vi "Check Length.vi"(7 "source vi name":string, 8 "error in (no error)":errorcluster, 9 "offset (0)":u64 format="%d bytes", 10 "length (-1: rest)":i64=-1 format="%d bytes", 11 "Pointer in":refnum<class "Pointer.lvclass">) -> (0 "error out":errorcluster, 1 "offset":u64 format="%d bytes", 2 "size":u64 format="%d bytes", 3 "Pointer out":refnum<class "Pointer.lvclass">)   [LabVIEW 2027, in "Memory Manager.lvlib" / "Pointer.lvclass"]
uses:
  Pointer.lvclass
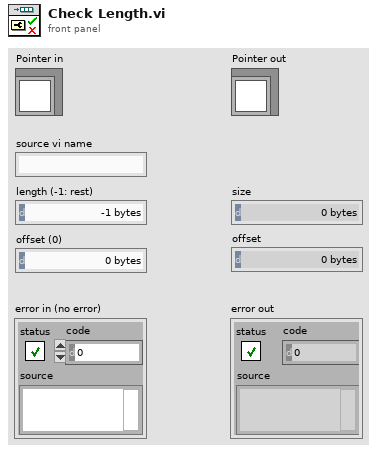
[diagram p1: front panel]
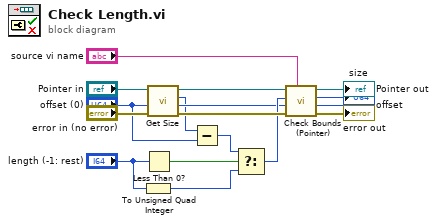
[diagram p0: block diagram]
diagram:
  n1 = To Unsigned Quad Integer(1:"length (-1: rest)") -> (0:w2:u64)
  n2 = Less Than 0?(x="length (-1: rest)") -> (x < 0?=w15:bool)
  n3 = call "Get Size.vi"("Pointer in"="Pointer in") -> ("size"=w1:u64, "Pointer out"=w12:refnum<class "Pointer.lvclass">)  [unwired: 9 in]
  n4 = Subtract(x=w1, y="offset (0)") -> (x-y=w3:u64)
  n5 = Select(t=w3, s=w15, f=w2) -> (s? t:f=w5:u64)
  n6 = call "Check Bounds (Pointer).vi"("source vi name"="source vi name", "error in (no error)"="error in (no error)", "offset (0)"="offset (0)", "size"=w5, "Pointer in"=w12) -> ("error out"=→"error out":errorcluster, "offset out"=→"offset":u64, "size"=→"size":u64, "Pointer out"=→"Pointer out":refnum<class "Pointer.lvclass">)  [unwired: 3 in]
